vi "AB_API Prepare Two Step Build.vi"(8 "error in (no error)":errorcluster, 10 "preview":bool, 11 "Build in":refnum<class "AB_Build.lvclass">) -> (0 "error out":errorcluster, 2 "Build Context":refnum<vi>, 3 "Class out":refnum<class "AB_Build.lvclass">)   [LabVIEW 2020]
uses:
  <vilib>/AppBuilder/AB_Classes/Build/AB_Build.lvclass
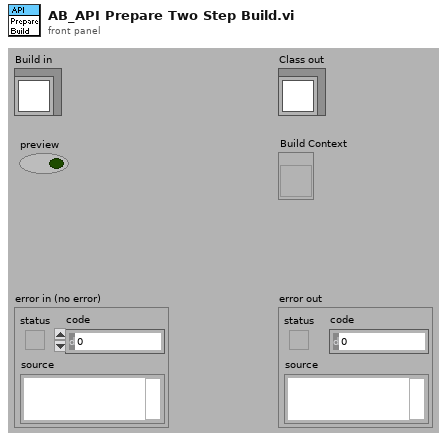
[diagram p1: front panel]
types:
  T1 = typedef "AB_Build.ctl" = cluster{"buildSpecName":string, "buildSpecDescription":string, "destinations":refnum<class "AB_Destination.lvclass">[], "exclusionOption":T2, "defaultLanguage":string, "supportedLanguages":string[], "excludedDirectories":path[], "buildContext":refnum<vi>, "buildObject":T3, "preview":bool, "programatic":bool, "progressBarEvents":T4, "userLog_Path":path, "preActionID":string, "preAction_Path":path, "postActionID":string, "postAction_Path":path, "eng_checkForBrokenVIs?":bool, "eng_verboseLinkerErrors?":bool, "localDest_Path":path, "targetDest_Path":path, "removeVIObject":u16, "cache":refnum<class "PreviewCache.lvclass">, "use cache":bool, "previewCache_ID":string, "buildCache_ID":string, "eng_TempLocalDest_Path":path, "eng_collectDependencies?":bool, "versionInfo":cluster{"buildVersion":cluster{"major":u16, "minor":u16, "patch":u16, "build":u16}, "autoIncrement":bool}, "eng_enableVIChecksums":bool}
  T2 = typedef "AB_Exclusion_Option.ctl" = cluster{"typedefs":bool, "polymorphicVIs":bool, "unusedLibraryItems":bool, "modifyLibraryFile":bool, "edit-timeDependencies":bool, "inlineVIs":bool, "dependent PPLs":bool, "dependent DLLs":bool}
  T3 = typedef "ItemRef.ctl" = u64
  T4 = typedef "provcom_ProgressBar_Events.ctl" = cluster{"newJob":refnum<user-event>, "newItem":refnum<user-event>, "errorMsg":T5, "cancel":refnum<user-event>}
  T5 = typedef "mxLvBuildError.ctl" = refnum<user-event>
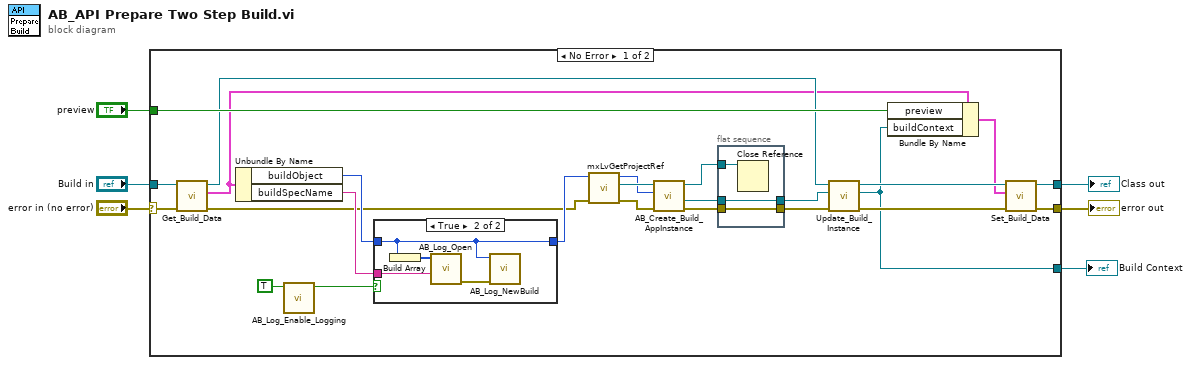
[diagram p0: block diagram]
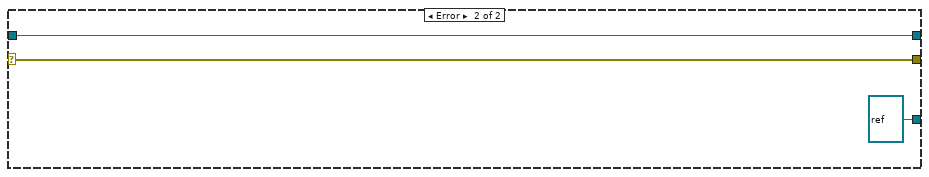
[diagram p3: hidden frame]
diagram:
  n1 = case shown="No Error" "error in (no error)" {
    selector: "error in (no error)" -> [w14 w42]
    tunnel: [w31 w42] -> w6
    tunnel: [w30 w41] -> w5
    tunnel: "preview" -> [w29 _]
    tunnel: "Build in" -> [w19 w41]
    tunnel: [w13 refnum<vi> refnum ("AppInstanceForBuild out")] -> w1
    frame No Error {
      n2 = call <vilib>:"Get_Build_Data.vi"("error in (no error)"=w14, "Class in"=w19) -> ("error out"=w16:errorcluster, "data"=w15:T1, "Class out"=w26:refnum<class "AB_Build.lvclass">)  [unwired: 7 out]
      n3 = Unbundle By Name(w15) -> ("buildObject"=w23:T3, "buildSpecName"=w20:string)
      n4 = call <vilib>:"AB_Log_Enable_Logging.vi"("read INI"=TRUE) -> ("log?"=w25:bool)  [unwired: 1 in, 9 out]
      n5 = case shown="True" w25 {
        tunnel: w23 -> [w35 w38]
        tunnel: [w35 w38] -> w24
        tunnel: w20 -> [_ w36]
        frame False {
        }
        frame True {
          n6 = Build Array(w38) -> (w39:T3[])
          n7 = call <vilib>:"AB_Log_Open.vi"("build spec name"=w36, "Objects"=w39) -> ("error out"=w37:errorcluster)  [unwired: 1 in, 8 out]
          n8 = call <vilib>:"AB_Log_NewBuild.vi"("error in (no error)"=w37, "Object"=w38) -> ()  [unwired: 10 out]
        }
      }
      n9 = call <resource>:"mxLvGetProjectRef.vi"("error in"=w16, "Item"=w24) -> ("error out"=w17:errorcluster, "Project Refnum"=w22:refnum<vi>, "Item"=w21:T3)  [unwired: 7 out]
      n10 = call <resource>:"AB_Create_Build_AppInstance.vi"("error in (no error)"=w17, "Object"=w21, "Project Refnum"=w22) -> ("error out"=w11:errorcluster, "Build app instance"=w9:refnum<vi>, "dup Project Refnum"=w12:refnum<vi>)  [unwired: 6 out]
      n11 = flat-sequence {
        tunnel: w12 -> [w34]
        tunnel: w11 -> [w33]
        tunnel: [w33] -> w10
        tunnel: [w32] -> w8
        tunnel: w9 -> [w32]
        frame #0 {
          n12 = Close Reference(reference=w34) -> ()  [unwired: 1 in, 1 out]
        }
      }
      n13 = call-dynamic "Update_Build_Instance.vi"("error in (no error)"=w10, "AppInstanceForBuild in"=w8, "Build in"=w26) -> ("error out"=w28:errorcluster, "AppInstanceForBuild out"=w13:refnum<vi>, "Build out"=w27:refnum<class "AB_Build.lvclass">)  [unwired: 6 out]
      n14 = Bundle By Name(cluster=w15, "preview"=w29, "buildContext"=w13) -> (w18:T1)
      n15 = call <vilib>:"Set_Build_Data.vi"("error in (no error)"=w28, "data"=w18, "Class in"=w27) -> ("error out"=w31:errorcluster, "Class out"=w30:refnum<class "AB_Build.lvclass">)  [unwired: 7 out]
    }
    frame Error {
    }
  }
  "error out" <- w6
  "Class out" <- w5
  "Build Context" <- w1
